vi "AutoCAD cmds NET.vi"(6 "AutoCAD cmd":T3, 7 "MathCAD results":T2, 8 "error in (no error)":errorcluster, 9 "path":path=path "C:/Documents and Settings/mw24/My Documents/Drawing2.dwg", 10 "Command":string="box 4 4 4\n_-view\n_swiso\n_shademode\nRealistic ") -> (0 "error out":errorcluster, 2 "IsQuiescent":bool)   [LabVIEW 2010]
uses:
  AutoCAD cmds.ctl
  MathCAD results ref.ctl
  Autodesk.AutoCAD.Interop
  Project commands.ctl
  AguaClara Library.lvlib
panel:
  out "error out 2":errorcluster
  out "Add":refnum<k24>
  in  "AcSaveAsType":T1(ring)
  out "new doc error":errorcluster
  out "Iterations":i32
  out "Visible":bool
  out "appended path":path
  out "basepath":string
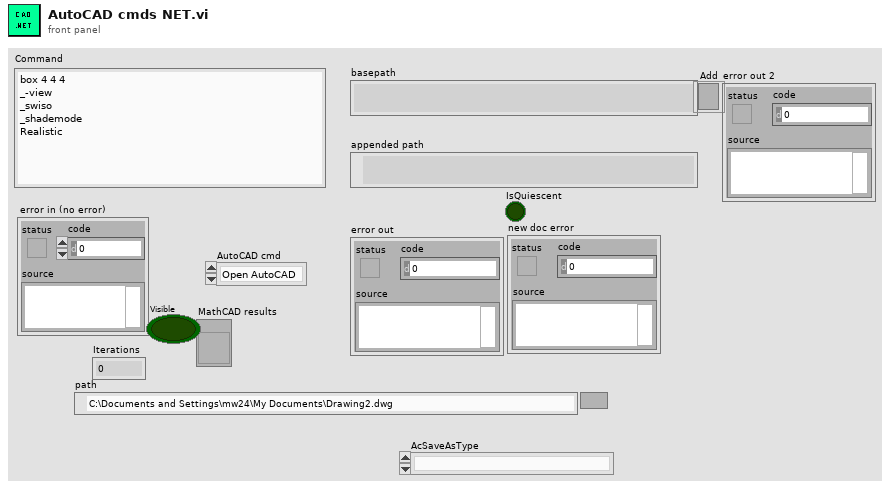
[diagram p1: front panel]
types:
  T1 = enum16{"", "acR14_dwg", "ac2000_dwg", "ac2000_dxf", "ac2000_Template", "ac2004_dwg", "ac2004_dxf", "ac2004_Template", "ac2007_dwg", "ac2007_dxf", "ac2007_Template", "acNative"}
  T2 = typedef "MathCAD results ref.ctl" = refnum<vi>
  T3 = typedef "AguaClara Library.lvlib/AutoCAD cmds.ctl" = enum16{"Open AutoCAD", "New Document", "Send Command", "Send Command Array", "Save picture", "Save File", "Close Doc", "Quit"}
  T4 = typedef "AguaClara Library.lvlib/Project commands.ctl" = enum16{"Load base file", "Load User", "Read paths", "Open Project", "New project", "Edit project", "Delete project", "Mail project", "save design", "open design"}
  T5 = cluster{"Label.Text":string, "Caption.Text":string[], "Control Type":u32, "Numeric":dbl, "Array":dbl[], "status":bool, "Outputs":bool[], "Str Array":string[], "String":string}[]
  T6 = typedef "AguaClara Library.lvlib/File paths.ctl" = cluster{"basepath":string, "AutoCAD script":string, "Design variables":string}
  T7 = typedef "AguaClara Library.lvlib/Project inputs.ctl" = cluster{"Project Name":string, "City":string, "State":string, "Country":string, "Notes":string}
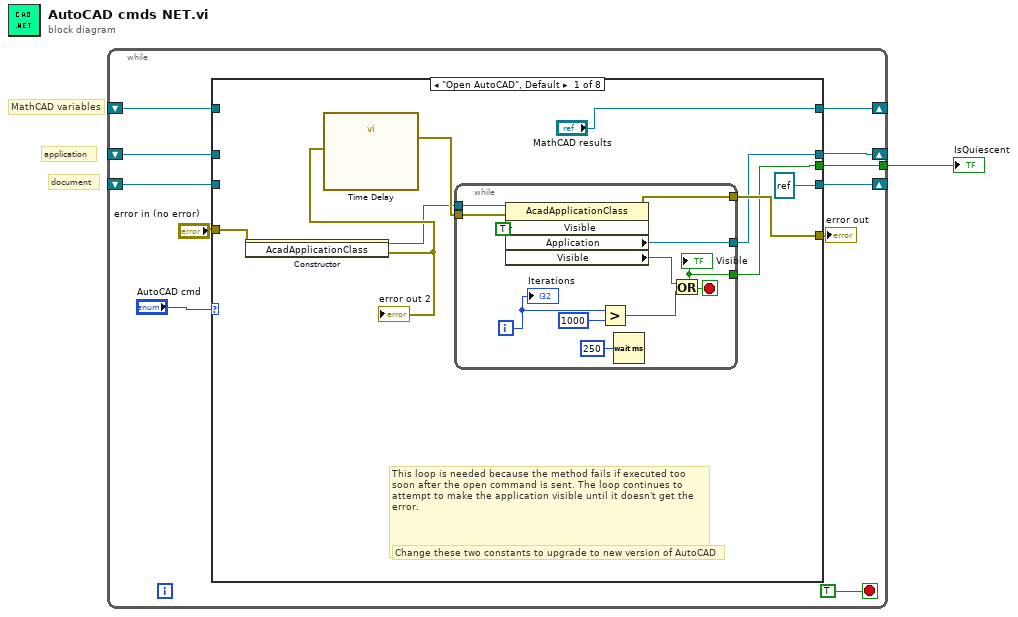
[diagram p0: block diagram]
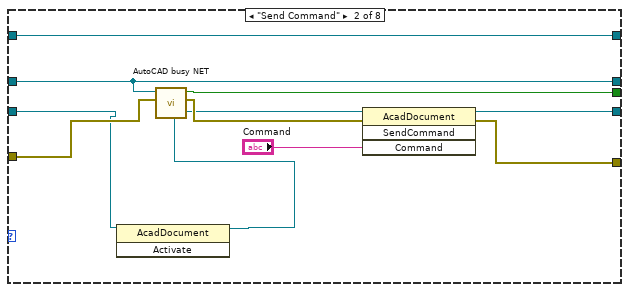
[diagram p2: hidden frame]
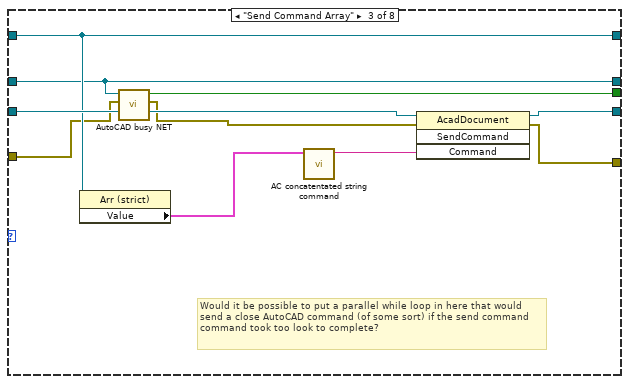
[diagram p3: hidden frame]
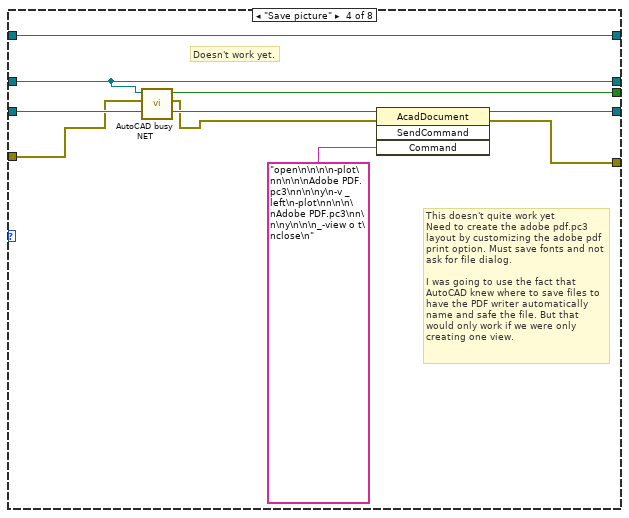
[diagram p4: hidden frame]
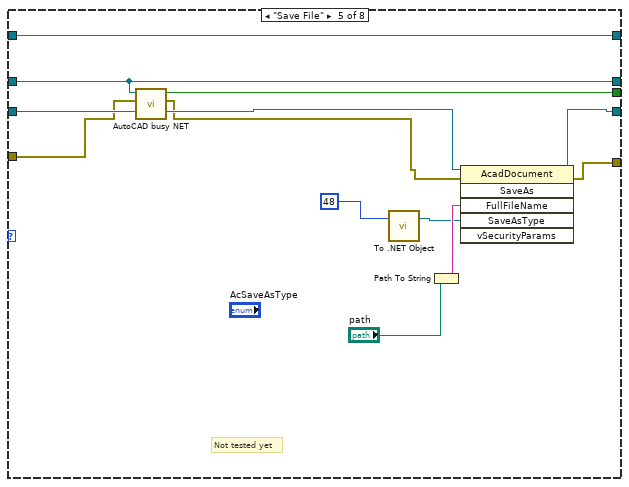
[diagram p5: hidden frame]
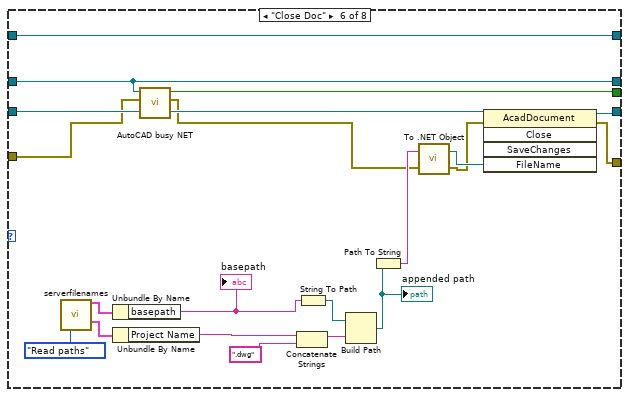
[diagram p6: hidden frame]
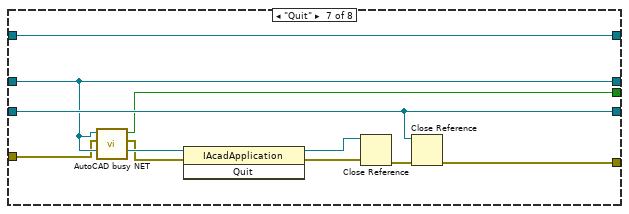
[diagram p7: hidden frame]
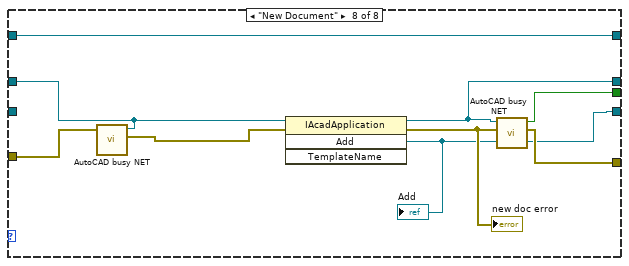
[diagram p8: hidden frame]
diagram:
  # "MathCAD variables"
  # "document"
  # "application"
  n1 = while {
    shift-right: [w11] -> _
    shift-left: _ -> [w6]
    shift-right: [w8] -> _
    shift-left: _ -> [w7]
    shift-right: [w4] -> _
    shift-left: _ -> [w3]
    tunnel: [w2] -> w1
    stop <- TRUE stop-if-true
    n2 = case shown="\"Open AutoCAD\", Default" "AutoCAD cmd" {
      tunnel: [w19 w38 w46 w56 w69 w80 w97 w109] -> w11
      tunnel: "error in (no error)" -> [w16 w37 w45 w55 w68 w79 w96 w110]
      tunnel: [w20 w40 w50 w60 w72 w91 w98 w108] -> w9
      tunnel: [refnum<k24> refnum ("Add") w41 w51 w58 w70 w92 w99 w104] -> w8
      tunnel: w7 -> [_ w34 w52 w59 w71 w93 w99 _]
      tunnel: w6 -> [_ w38 w46 w56 w69 w80 w97 w111]
      tunnel: ["MathCAD results" w39 w49 w61 w73 w81 w103 w112] -> w4
      tunnel: w3 -> [_ w39 w49 w61 w73 w81 w103 w112]
      tunnel: [w18 w35 w43 w53 w66 w78 w94 w107] -> w2
      frame "Open AutoCAD", Default {
        # "This loop is needed because the method fails if executed too soon after the open command is sent. The loop continues to attempt to make the application visible until it doesn't get the error."
        # "Change these two constants to upgrade to new version of AutoCAD"
        n3 = constructor class="AcadApplicationClass"(error in=w16) -> (reference out=w14:refnum<k24>, error out=w15:errorcluster)  [unwired: 2 in, 1 out]
        "error out 2" <- w15
        n4 = call "Time Delay"("error in (no error)"=w15) -> ("error out"=w17:errorcluster)  [unwired: 10 in]
        n5 = while {
          tunnel: w14 -> [w32]
          tunnel: w17 -> [w31]
          tunnel: [w26] -> w20
          tunnel: [w23] -> w19
          tunnel: [w24] -> w18
          i -> [w29]
          stop <- w30 stop-if-true
          n6 = property class="AcadApplicationClass"(reference=w32, error in=w31, "Visible"=TRUE) -> (error out=w26:errorcluster, "Application"=w23:refnum<k24>, "Visible"=w24:bool)  [unwired: 1 out]
          "Visible" <- w24
          n7 = Greater?(x=w29, y=1000) -> (0:w27:bool)
          n8 = Wait (ms)(milliseconds to wait=u32 250) -> ()  [unwired: 1 out]
          n9 = Or(x=w24, y=w27) -> (x .or. y?=w30:bool)
          "Iterations" <- w29
        }
      }
      frame "Send Command" {
        n10 = invoke class="AcadDocument" method="Activate"(reference=w34) -> (reference out=w33:refnum<k24>)  [unwired: 2 in, 2 out]
        n11 = call "AutoCAD busy NET.vi"("error in (no error)"=w37, "Application 2"=w38) -> ("error out"=w36:errorcluster, "IsQuiescent"=w35:bool)  [unwired: 4 in]
        n12 = invoke class="AcadDocument" method="SendCommand"(reference=w33, error in=w36, "Command"="Command") -> (reference out=w41:refnum<k24>, error out=w40:errorcluster)  [unwired: 1 in, 2 out]
      }
      frame "Send Command Array" {
        # "Would it be possible to put a parallel while loop in here that would send a close AutoCAD command (of some sort) if the send command command took too look to complete?"
        n13 = property class="Arr (strict)"(reference=w49) -> ("Value"=w48:T5)  [unwired: 1 in, 2 out]
        n14 = call "AutoCAD busy NET.vi"("error in (no error)"=w45, "Application 2"=w46) -> ("error out"=w44:errorcluster, "IsQuiescent"=w43:bool)  [unwired: 4 in]
        n15 = call "AC concatentated string command.vi"("MathCAD results"=w48) -> ("AC concatenated string"=w47:string)  [unwired: 9 in, 1 out]
        n16 = invoke class="AcadDocument" method="SendCommand"(reference=w52, error in=w44, "Command"=w47) -> (reference out=w51:refnum<k24>, error out=w50:errorcluster)  [unwired: 1 in, 2 out]
      }
      frame "Save picture" {
        # "Doesn't work yet."
        # "This doesn't quite work yet\nNeed to create the adobe pdf.pc3 layout by customizing the adobe pdf print option. Must save fonts and not ask for file dialog.\n\nI was going to use the fact that AutoCAD knew where to save files to have the PDF writer automatically name and safe the file. But that would only work if we were only creating one view."
        n17 = call "AutoCAD busy NET.vi"("error in (no error)"=w55, "Application 2"=w56) -> ("error out"=w54:errorcluster, "IsQuiescent"=w53:bool)  [unwired: 4 in]
        n18 = invoke class="AcadDocument" method="SendCommand"(reference=w59, error in=w54, "Command"="open\n\n\n\n-plot\nn\n\n\nAdobe PDF.pc3\nn\n\ny\n-v _left\n-plot\nn\n\n\nAdobe PDF.pc3\nn\n\ny\n\n\n_-view o t\nclose\n") -> (reference out=w58:refnum<k24>, error out=w60:errorcluster)  [unwired: 1 in, 2 out]
      }
      frame "Save File" {
        # "Not tested yet"
        n19 = call "AutoCAD busy NET.vi"("error in (no error)"=w68, "Application 2"=w69) -> ("error out"=w67:errorcluster, "IsQuiescent"=w66:bool)  [unwired: 4 in]
        n20 = call <vilib>:"To .NET Object.vi"("anything"=i8 48) -> (".NET object"=w62:refnum<k24>)  [unwired: 1 in, 1 out]
        n21 = Path To String(path="path") -> (string=w64:string)
        n22 = invoke class="AcadDocument" method="SaveAs"(reference=w71, error in=w67, "FullFileName"=w64, "SaveAsType"=w62) -> (reference out=w70:refnum<k24>, error out=w72:errorcluster)  [unwired: 2 in, 4 out]
      }
      frame "Close Doc" {
        n23 = call "serverfilenames.vi"("Project command"=Project_commands."Read paths") -> ("File paths"=w88:T6, "Project Info out"=w89:T7)  [unwired: 10 in, 3 out]
        n24 = Unbundle By Name(w88) -> ("basepath"=w86:string)
        "basepath" <- w86
        n25 = Unbundle By Name(w89) -> ("Project Name"=w90:string)
        n26 = call "AutoCAD busy NET.vi"("error in (no error)"=w79, "Application 2"=w80) -> ("error out"=w75:errorcluster, "IsQuiescent"=w78:bool)  [unwired: 4 in]
        n27 = Concatenate Strings(w90, ".dwg" ("string")) -> (w83:string)
        n28 = String To Path(string=w86) -> (path=w85:path)
        n29 = Build Path(base path=w85, name or relative path=w83) -> (appended path=w84:path)
        "appended path" <- w84
        n30 = Path To String(path=w84) -> (string=w76:string)
        n31 = call <vilib>:"To .NET Object.vi"("error in (no error)"=w75, "anything"=w76) -> ("error out"=w74:errorcluster, ".NET object"=w77:refnum<k24>)
        n32 = invoke class="AcadDocument" method="Close"(reference=w93, error in=w74, "FileName"=w77) -> (reference out=w92:refnum<k24>, error out=w91:errorcluster)  [unwired: 2 in, 3 out]
      }
      frame "Quit" {
        n33 = call "AutoCAD busy NET.vi"("error in (no error)"=w96, "Application 2"=w97) -> ("error out"=w95:errorcluster, "IsQuiescent"=w94:bool)  [unwired: 4 in]
        n34 = invoke class="IAcadApplication" method="Quit"(reference=w97, error in=w95) -> (reference out=w102:refnum<k24>, error out=w101:errorcluster)  [unwired: 1 in, 1 out]
        n35 = Close Reference(reference=w102, error in (no error)=w101) -> (error out=w100:errorcluster)
        n36 = Close Reference(reference=w99, error in (no error)=w100) -> (error out=w98:errorcluster)
      }
      frame "New Document" {
        n37 = call "AutoCAD busy NET.vi"("error in (no error)"=w110, "Application 2"=w111) -> ("error out"=w105:errorcluster)  [unwired: 4 in, 1 out]
        n38 = invoke class="IAcadApplication" method="Add"(reference=w111, error in=w105) -> (reference out=w109:refnum<k24>, error out=w106:errorcluster, "Add"=w104:refnum<k24>)  [unwired: 2 in, 1 out]
        "new doc error" <- w106
        "Add" <- w104
        n39 = call "AutoCAD busy NET.vi"("error in (no error)"=w106, "Application 2"=w109) -> ("error out"=w108:errorcluster, "IsQuiescent"=w107:bool)  [unwired: 4 in]
      }
    }
    "error out" <- w9
  }
  "IsQuiescent" <- w1
